vi "Lab Panel V5.10.vi"() -> ()   [LabVIEW 2013] (continued)
                      tunnel: w2159 -> [w2170 w2172 _]
                      tunnel: ["CHART PASS" "CYCLE PASS" "T-RISE PASS"] -> w2163
                      frame "CHART TEST", Default {
                      }
                      frame "CYCLE TEST" {
                      }
                      frame "T-RISE TEST" {
                      }
                    }
                    n1123 = Increment(x=w2159) -> (x+1=w2160:dbl)
                    n1124 = Greater Or Equal?(x=w2167, y=w2160) -> (x >= y?=w2169:bool)
                    n1125 = case shown="True" w2169 {
                      tunnel: w2164 -> [w2179 _]
                      tunnel: w2163 -> [w2178 _]
                      tunnel: w2162 -> [w2177 _]
                      tunnel: w2161 -> [w2176 _]
                      frame True {
                        n1126 = stacked-sequence {
                          tunnel: w2179 -> [w2183 _]
                          tunnel: w2178 -> [w2181 w2187]
                          tunnel: w2177 -> [_ w2190]
                          tunnel: w2176 -> [w2180 _]
                          frame #0 {
                            n1127 = Build Array(w2181) -> (w2184:string[])
                            n1128 = Build Array(w2183) -> (w2182:dbl[])
                            n1129 = TDMS Write(0:w2180, 5:"TEST PASS", 7:w2184, 9:w2182) -> (15:w2186:errorcluster)  [unwired: 2 in, 3 out]
                            n1130 = local write "data file error"(w2186) -> ()
                          }
                          frame #1 {
                            n1131 = Bundle(cluster=w2190, "STATUS"=w2187) -> (w2188:T4)  [unwired: 2 in]
                            n1132 = local write "RESULT LAB02-1"(TRUE) -> ()
                            n1133 = local write "DISP LAB02-1"(w2188) -> ()
                          }
                        }
                      }
                      frame False {
                      }
                    }
                  }
                }
              }
              frame #3 {
                # "LAB02-2"
                n1134 = Less?(x=w2191, y=2) -> (x < y?=w2194:bool)
                n1135 = local read "DISP LAB02-2"() -> (w2196:T4)
                n1136 = Unbundle(w2196) -> ("STATUS"=w2197:string)  [unwired: 2 out]
                n1137 = Equal?(x=w2197, y="RUN") -> (x = y?=w2193:bool)
                n1138 = And(x=w2193, y=w2194) -> (x .and. y?=w2192:bool)
                n1139 = case shown="True" w2192 {
                  tunnel: w2196 -> [_ w2202]
                  tunnel: w2191 -> [_ w2206]
                  frame False {
                  }
                  frame True {
                    n1140 = local read "SET LAB02-2"() -> (w2208:T5)
                    n1141 = local read "TDMS LAB02-2"() -> (w2201:refnum<k34>)
                    n1142 = Unbundle(w2202) -> ("CYCLE"=w2207:dbl)  [unwired: 2 out]
                    n1143 = Unbundle(w2208) -> ("CYCLES"=w2199:dbl, "T-RISE mins"=w2205:dbl)  [unwired: 3 out]
                    n1144 = case shown="\"T-RISE TEST\"" w2206 {
                      tunnel: w2205 -> [_ _ w2215]
                      tunnel: [w2210 w2212 w2215] -> w2204
                      tunnel: w2199 -> [w2210 w2212 _]
                      tunnel: ["CHART PASS" "CYCLE PASS" "T-RISE PASS"] -> w2203
                      frame "CHART TEST", Default {
                      }
                      frame "CYCLE TEST" {
                      }
                      frame "T-RISE TEST" {
                      }
                    }
                    n1145 = Increment(x=w2199) -> (x+1=w2200:dbl)
                    n1146 = Greater Or Equal?(x=w2207, y=w2200) -> (x >= y?=w2209:bool)
                    n1147 = case shown="True" w2209 {
                      tunnel: w2204 -> [w2219 _]
                      tunnel: w2203 -> [w2218 _]
                      tunnel: w2202 -> [w2217 _]
                      tunnel: w2201 -> [w2216 _]
                      frame True {
                        n1148 = stacked-sequence {
                          tunnel: w2219 -> [w2223 _]
                          tunnel: w2218 -> [w2221 w2227]
                          tunnel: w2217 -> [_ w2230]
                          tunnel: w2216 -> [w2220 _]
                          frame #0 {
                            n1149 = Build Array(w2221) -> (w2224:string[])
                            n1150 = Build Array(w2223) -> (w2222:dbl[])
                            n1151 = TDMS Write(0:w2220, 5:"TEST PASS", 7:w2224, 9:w2222) -> (15:w2226:errorcluster)  [unwired: 2 in, 3 out]
                            n1152 = local write "data file error"(w2226) -> ()
                          }
                          frame #1 {
                            n1153 = Bundle(cluster=w2230, "STATUS"=w2227) -> (w2228:T4)  [unwired: 2 in]
                            n1154 = local write "RESULT LAB02-2"(TRUE) -> ()
                            n1155 = local write "DISP LAB02-2"(w2228) -> ()
                          }
                        }
                      }
                      frame False {
                      }
                    }
                  }
                }
              }
              frame #4 {
                # "LAB03-1"
                n1156 = Less?(x=w2231, y=2) -> (x < y?=w2234:bool)
                n1157 = local read "DISP LAB03-1"() -> (w2236:T4)
                n1158 = Unbundle(w2236) -> ("STATUS"=w2237:string)  [unwired: 2 out]
                n1159 = Equal?(x=w2237, y="RUN") -> (x = y?=w2233:bool)
                n1160 = And(x=w2233, y=w2234) -> (x .and. y?=w2232:bool)
                n1161 = case shown="True" w2232 {
                  tunnel: w2236 -> [_ w2242]
                  tunnel: w2231 -> [_ w2246]
                  frame False {
                  }
                  frame True {
                    n1162 = local read "SET LAB03-1"() -> (w2248:T5)
                    n1163 = local read "TDMS LAB03-1"() -> (w2241:refnum<k34>)
                    n1164 = Unbundle(w2242) -> ("CYCLE"=w2247:dbl)  [unwired: 2 out]
                    n1165 = Unbundle(w2248) -> ("CYCLES"=w2239:dbl, "T-RISE mins"=w2245:dbl)  [unwired: 3 out]
                    n1166 = case shown="\"T-RISE TEST\"" w2246 {
                      tunnel: w2245 -> [_ _ w2255]
                      tunnel: [w2250 w2252 w2255] -> w2244
                      tunnel: w2239 -> [w2250 w2252 _]
                      tunnel: ["CHART PASS" "CYCLE PASS" "T-RISE PASS"] -> w2243
                      frame "CHART TEST", Default {
                      }
                      frame "CYCLE TEST" {
                      }
                      frame "T-RISE TEST" {
                      }
                    }
                    n1167 = Increment(x=w2239) -> (x+1=w2240:dbl)
                    n1168 = Greater Or Equal?(x=w2247, y=w2240) -> (x >= y?=w2249:bool)
                    n1169 = case shown="True" w2249 {
                      tunnel: w2244 -> [w2259 _]
                      tunnel: w2243 -> [w2258 _]
                      tunnel: w2242 -> [w2257 _]
                      tunnel: w2241 -> [w2256 _]
                      frame True {
                        n1170 = stacked-sequence {
                          tunnel: w2259 -> [w2263 _]
                          tunnel: w2258 -> [w2261 w2267]
                          tunnel: w2257 -> [_ w2270]
                          tunnel: w2256 -> [w2260 _]
                          frame #0 {
                            n1171 = Build Array(w2261) -> (w2264:string[])
                            n1172 = Build Array(w2263) -> (w2262:dbl[])
                            n1173 = TDMS Write(0:w2260, 5:"TEST PASS", 7:w2264, 9:w2262) -> (15:w2266:errorcluster)  [unwired: 2 in, 3 out]
                            n1174 = local write "data file error"(w2266) -> ()
                          }
                          frame #1 {
                            n1175 = Bundle(cluster=w2270, "STATUS"=w2267) -> (w2268:T4)  [unwired: 2 in]
                            n1176 = local write "RESULT LAB03-1"(TRUE) -> ()
                            n1177 = local write "DISP LAB03-1"(w2268) -> ()
                          }
                        }
                      }
                      frame False {
                      }
                    }
                  }
                }
              }
              frame #5 {
                # "LAB03-2"
                n1178 = Less?(x=w2271, y=2) -> (x < y?=w2274:bool)
                n1179 = local read "DISP LAB03-2"() -> (w2276:T4)
                n1180 = Unbundle(w2276) -> ("STATUS"=w2277:string)  [unwired: 2 out]
                n1181 = Equal?(x=w2277, y="RUN") -> (x = y?=w2273:bool)
                n1182 = And(x=w2273, y=w2274) -> (x .and. y?=w2272:bool)
                n1183 = case shown="True" w2272 {
                  tunnel: w2276 -> [_ w2282]
                  tunnel: w2271 -> [_ w2286]
                  frame False {
                  }
                  frame True {
                    n1184 = local read "SET LAB03-2"() -> (w2288:T5)
                    n1185 = local read "TDMS LAB03-2"() -> (w2281:refnum<k34>)
                    n1186 = Unbundle(w2282) -> ("CYCLE"=w2287:dbl)  [unwired: 2 out]
                    n1187 = Unbundle(w2288) -> ("CYCLES"=w2279:dbl, "T-RISE mins"=w2285:dbl)  [unwired: 3 out]
                    n1188 = case shown="\"T-RISE TEST\"" w2286 {
                      tunnel: w2285 -> [_ _ w2295]
                      tunnel: [w2290 w2292 w2295] -> w2284
                      tunnel: w2279 -> [w2290 w2292 _]
                      tunnel: ["CHART PASS" "CYCLE PASS" "T-RISE PASS"] -> w2283
                      frame "CHART TEST", Default {
                      }
                      frame "CYCLE TEST" {
                      }
                      frame "T-RISE TEST" {
                      }
                    }
                    n1189 = Increment(x=w2279) -> (x+1=w2280:dbl)
                    n1190 = Greater Or Equal?(x=w2287, y=w2280) -> (x >= y?=w2289:bool)
                    n1191 = case shown="True" w2289 {
                      tunnel: w2284 -> [w2299 _]
                      tunnel: w2283 -> [w2298 _]
                      tunnel: w2282 -> [w2297 _]
                      tunnel: w2281 -> [w2296 _]
                      frame True {
                        n1192 = stacked-sequence {
                          tunnel: w2299 -> [w2303 _]
                          tunnel: w2298 -> [w2301 w2307]
                          tunnel: w2297 -> [_ w2310]
                          tunnel: w2296 -> [w2300 _]
                          frame #0 {
                            n1193 = Build Array(w2301) -> (w2304:string[])
                            n1194 = Build Array(w2303) -> (w2302:dbl[])
                            n1195 = TDMS Write(0:w2300, 5:"TEST PASS", 7:w2304, 9:w2302) -> (15:w2306:errorcluster)  [unwired: 2 in, 3 out]
                            n1196 = local write "data file error"(w2306) -> ()
                          }
                          frame #1 {
                            n1197 = Bundle(cluster=w2310, "STATUS"=w2307) -> (w2308:T4)  [unwired: 2 in]
                            n1198 = local write "RESULT LAB03-2"(TRUE) -> ()
                            n1199 = local write "DISP LAB03-2"(w2308) -> ()
                          }
                        }
                      }
                      frame False {
                      }
                    }
                  }
                }
              }
              frame #6 {
                # "LAB04-1"
                n1200 = Less?(x=w2311, y=2) -> (x < y?=w2314:bool)
                n1201 = local read "DISP LAB04-1"() -> (w2316:T4)
                n1202 = Unbundle(w2316) -> ("STATUS"=w2317:string)  [unwired: 2 out]
                n1203 = Equal?(x=w2317, y="RUN") -> (x = y?=w2313:bool)
                n1204 = And(x=w2313, y=w2314) -> (x .and. y?=w2312:bool)
                n1205 = case shown="True" w2312 {
                  tunnel: w2316 -> [_ w2322]
                  tunnel: w2311 -> [_ w2326]
                  frame False {
                  }
                  frame True {
                    n1206 = local read "SET LAB04-1"() -> (w2328:T5)
                    n1207 = local read "TDMS LAB04-1"() -> (w2321:refnum<k34>)
                    n1208 = Unbundle(w2322) -> ("CYCLE"=w2327:dbl)  [unwired: 2 out]
                    n1209 = Unbundle(w2328) -> ("CYCLES"=w2319:dbl, "T-RISE mins"=w2325:dbl)  [unwired: 3 out]
                    n1210 = case shown="\"T-RISE TEST\"" w2326 {
                      tunnel: w2325 -> [_ _ w2335]
                      tunnel: [w2330 w2332 w2335] -> w2324
                      tunnel: w2319 -> [w2330 w2332 _]
                      tunnel: ["CHART PASS" "CYCLE PASS" "T-RISE PASS"] -> w2323
                      frame "CHART TEST", Default {
                      }
                      frame "CYCLE TEST" {
                      }
                      frame "T-RISE TEST" {
                      }
                    }
                    n1211 = Increment(x=w2319) -> (x+1=w2320:dbl)
                    n1212 = Greater Or Equal?(x=w2327, y=w2320) -> (x >= y?=w2329:bool)
                    n1213 = case shown="True" w2329 {
                      tunnel: w2324 -> [w2339 _]
                      tunnel: w2323 -> [w2338 _]
                      tunnel: w2322 -> [w2337 _]
                      tunnel: w2321 -> [w2336 _]
                      frame True {
                        n1214 = stacked-sequence {
                          tunnel: w2339 -> [w2343 _]
                          tunnel: w2338 -> [w2341 w2347]
                          tunnel: w2337 -> [_ w2350]
                          tunnel: w2336 -> [w2340 _]
                          frame #0 {
                            n1215 = Build Array(w2341) -> (w2344:string[])
                            n1216 = Build Array(w2343) -> (w2342:dbl[])
                            n1217 = TDMS Write(0:w2340, 5:"TEST PASS", 7:w2344, 9:w2342) -> (15:w2346:errorcluster)  [unwired: 2 in, 3 out]
                            n1218 = local write "data file error"(w2346) -> ()
                          }
                          frame #1 {
                            n1219 = Bundle(cluster=w2350, "STATUS"=w2347) -> (w2348:T4)  [unwired: 2 in]
                            n1220 = local write "RESULT LAB04-1"(TRUE) -> ()
                            n1221 = local write "DISP LAB04-1"(w2348) -> ()
                          }
                        }
                      }
                      frame False {
                      }
                    }
                  }
                }
              }
              frame #7 {
                # "LAB04-2"
                n1222 = Less?(x=w2351, y=2) -> (x < y?=w2354:bool)
                n1223 = local read "DISP LAB04-2"() -> (w2356:T4)
                n1224 = Unbundle(w2356) -> ("STATUS"=w2357:string)  [unwired: 2 out]
                n1225 = Equal?(x=w2357, y="RUN") -> (x = y?=w2353:bool)
                n1226 = And(x=w2353, y=w2354) -> (x .and. y?=w2352:bool)
                n1227 = case shown="True" w2352 {
                  tunnel: w2356 -> [_ w2362]
                  tunnel: w2351 -> [_ w2366]
                  frame False {
                  }
                  frame True {
                    n1228 = local read "SET LAB04-2"() -> (w2368:T5)
                    n1229 = local read "TDMS LAB04-2"() -> (w2361:refnum<k34>)
                    n1230 = Unbundle(w2362) -> ("CYCLE"=w2367:dbl)  [unwired: 2 out]
                    n1231 = Unbundle(w2368) -> ("CYCLES"=w2359:dbl, "T-RISE mins"=w2365:dbl)  [unwired: 3 out]
                    n1232 = case shown="\"T-RISE TEST\"" w2366 {
                      tunnel: w2365 -> [_ _ w2375]
                      tunnel: [w2370 w2372 w2375] -> w2364
                      tunnel: w2359 -> [w2370 w2372 _]
                      tunnel: ["CHART PASS" "CYCLE PASS" "T-RISE PASS"] -> w2363
                      frame "CHART TEST", Default {
                      }
                      frame "CYCLE TEST" {
                      }
                      frame "T-RISE TEST" {
                      }
                    }
                    n1233 = Increment(x=w2359) -> (x+1=w2360:dbl)
                    n1234 = Greater Or Equal?(x=w2367, y=w2360) -> (x >= y?=w2369:bool)
                    n1235 = case shown="True" w2369 {
                      tunnel: w2364 -> [w2379 _]
                      tunnel: w2363 -> [w2378 _]
                      tunnel: w2362 -> [w2377 _]
                      tunnel: w2361 -> [w2376 _]
                      frame True {
                        n1236 = stacked-sequence {
                          tunnel: w2379 -> [w2383 _]
                          tunnel: w2378 -> [w2381 w2387]
                          tunnel: w2377 -> [_ w2390]
                          tunnel: w2376 -> [w2380 _]
                          frame #0 {
                            n1237 = Build Array(w2381) -> (w2384:string[])
                            n1238 = Build Array(w2383) -> (w2382:dbl[])
                            n1239 = TDMS Write(0:w2380, 5:"TEST PASS", 7:w2384, 9:w2382) -> (15:w2386:errorcluster)  [unwired: 2 in, 3 out]
                            n1240 = local write "data file error"(w2386) -> ()
                          }
                          frame #1 {
                            n1241 = Bundle(cluster=w2390, "STATUS"=w2387) -> (w2388:T4)  [unwired: 2 in]
                            n1242 = local write "RESULT LAB04-2"(TRUE) -> ()
                            n1243 = local write "DISP LAB04-2"(w2388) -> ()
                          }
                        }
                      }
                      frame False {
                      }
                    }
                  }
                }
              }
              frame #8 {
                # "LAB05-1"
                n1244 = Less?(x=w2391, y=2) -> (x < y?=w2394:bool)
                n1245 = local read "DISP LAB05-1"() -> (w2396:T4)
                n1246 = Unbundle(w2396) -> ("STATUS"=w2397:string)  [unwired: 2 out]
                n1247 = Equal?(x=w2397, y="RUN") -> (x = y?=w2393:bool)
                n1248 = And(x=w2393, y=w2394) -> (x .and. y?=w2392:bool)
                n1249 = case shown="True" w2392 {
                  tunnel: w2396 -> [_ w2402]
                  tunnel: w2391 -> [_ w2406]
                  frame False {
                  }
                  frame True {
                    n1250 = local read "SET LAB05-1"() -> (w2408:T5)
                    n1251 = local read "TDMS LAB05-1"() -> (w2401:refnum<k34>)
                    n1252 = Unbundle(w2402) -> ("CYCLE"=w2407:dbl)  [unwired: 2 out]
                    n1253 = Unbundle(w2408) -> ("CYCLES"=w2399:dbl, "T-RISE mins"=w2405:dbl)  [unwired: 3 out]
                    n1254 = case shown="\"T-RISE TEST\"" w2406 {
                      tunnel: w2405 -> [_ _ w2415]
                      tunnel: [w2410 w2412 w2415] -> w2404
                      tunnel: w2399 -> [w2410 w2412 _]
                      tunnel: ["CHART PASS" "CYCLE PASS" "T-RISE PASS"] -> w2403
                      frame "CHART TEST", Default {
                      }
                      frame "CYCLE TEST" {
                      }
                      frame "T-RISE TEST" {
                      }
                    }
                    n1255 = Increment(x=w2399) -> (x+1=w2400:dbl)
                    n1256 = Greater Or Equal?(x=w2407, y=w2400) -> (x >= y?=w2409:bool)
                    n1257 = case shown="True" w2409 {
                      tunnel: w2404 -> [w2419 _]
                      tunnel: w2403 -> [w2418 _]
                      tunnel: w2402 -> [w2417 _]
                      tunnel: w2401 -> [w2416 _]
                      frame True {
                        n1258 = stacked-sequence {
                          tunnel: w2419 -> [w2423 _]
                          tunnel: w2418 -> [w2421 w2427]
                          tunnel: w2417 -> [_ w2430]
                          tunnel: w2416 -> [w2420 _]
                          frame #0 {
                            n1259 = Build Array(w2421) -> (w2424:string[])
                            n1260 = Build Array(w2423) -> (w2422:dbl[])
                            n1261 = TDMS Write(0:w2420, 5:"TEST PASS", 7:w2424, 9:w2422) -> (15:w2426:errorcluster)  [unwired: 2 in, 3 out]
                            n1262 = local write "data file error"(w2426) -> ()
                          }
                          frame #1 {
                            n1263 = Bundle(cluster=w2430, "STATUS"=w2427) -> (w2428:T4)  [unwired: 2 in]
                            n1264 = local write "RESULT LAB05-1"(TRUE) -> ()
                            n1265 = local write "DISP LAB05-1"(w2428) -> ()
                          }
                        }
                      }
                      frame False {
                      }
                    }
                  }
                }
              }
              frame #9 {
                # "LAB05-2"
                n1266 = Less?(x=w2431, y=2) -> (x < y?=w2434:bool)
                n1267 = local read "DISP LAB05-2"() -> (w2436:T4)
                n1268 = Unbundle(w2436) -> ("STATUS"=w2437:string)  [unwired: 2 out]
                n1269 = Equal?(x=w2437, y="RUN") -> (x = y?=w2433:bool)
                n1270 = And(x=w2433, y=w2434) -> (x .and. y?=w2432:bool)
                n1271 = case shown="True" w2432 {
                  tunnel: w2436 -> [_ w2442]
                  tunnel: w2431 -> [_ w2446]
                  frame False {
                  }
                  frame True {
                    n1272 = local read "SET LAB05-2"() -> (w2448:T5)
                    n1273 = local read "TDMS LAB05-2"() -> (w2441:refnum<k34>)
                    n1274 = Unbundle(w2442) -> ("CYCLE"=w2447:dbl)  [unwired: 2 out]
                    n1275 = Unbundle(w2448) -> ("CYCLES"=w2439:dbl, "T-RISE mins"=w2445:dbl)  [unwired: 3 out]
                    n1276 = case shown="\"T-RISE TEST\"" w2446 {
                      tunnel: w2445 -> [_ _ w2455]
                      tunnel: [w2450 w2452 w2455] -> w2444
                      tunnel: w2439 -> [w2450 w2452 _]
                      tunnel: ["CHART PASS" "CYCLE PASS" "T-RISE PASS"] -> w2443
                      frame "CHART TEST", Default {
                      }
                      frame "CYCLE TEST" {
                      }
                      frame "T-RISE TEST" {
                      }
                    }
                    n1277 = Increment(x=w2439) -> (x+1=w2440:dbl)
                    n1278 = Greater Or Equal?(x=w2447, y=w2440) -> (x >= y?=w2449:bool)
                    n1279 = case shown="True" w2449 {
                      tunnel: w2444 -> [w2459 _]
                      tunnel: w2443 -> [w2458 _]
                      tunnel: w2442 -> [w2457 _]
                      tunnel: w2441 -> [w2456 _]
                      frame True {
                        n1280 = stacked-sequence {
                          tunnel: w2459 -> [w2463 _]
                          tunnel: w2458 -> [w2461 w2467]
                          tunnel: w2457 -> [_ w2470]
                          tunnel: w2456 -> [w2460 _]
                          frame #0 {
                            n1281 = Build Array(w2461) -> (w2464:string[])
                            n1282 = Build Array(w2463) -> (w2462:dbl[])
                            n1283 = TDMS Write(0:w2460, 5:"TEST PASS", 7:w2464, 9:w2462) -> (15:w2466:errorcluster)  [unwired: 2 in, 3 out]
                            n1284 = local write "data file error"(w2466) -> ()
                          }
                          frame #1 {
                            n1285 = Bundle(cluster=w2470, "STATUS"=w2467) -> (w2468:T4)  [unwired: 2 in]
                            n1286 = local write "RESULT LAB05-2"(TRUE) -> ()
                            n1287 = local write "DISP LAB05-2"(w2468) -> ()
                          }
                        }
                      }
                      frame False {
                      }
                    }
                  }
                }
              }
            }
          }
          frame #5 {
            # "check if test cycles reached for temperature rise test"
            n1288 = stacked-sequence {
              tunnel: w2500 -> [_ _ _ _ _ _ _ _ _ _]
              tunnel: w2499 -> [_ _ _ _ _ _ _ _ _ _]
              tunnel: w2498 -> [_ _ _ _ _ _ _ _ _ _]
              tunnel: w2497 -> [_ _ _ _ _ _ _ _ _ _]
              tunnel: w2496 -> [_ _ _ _ _ _ _ _ _ _]
              tunnel: w2495 -> [_ _ _ _ _ _ _ _ _ _]
              tunnel: w2494 -> [_ _ _ _ _ _ _ _ _ _]
              tunnel: w2493 -> [_ _ _ _ _ _ _ _ _ _]
              tunnel: w2492 -> [_ _ _ _ _ _ _ _ _ _]
              tunnel: w2491 -> [_ _ _ _ _ _ _ _ _ _]
              tunnel: w2490 -> [w2506 _ _ _ _ _ _ _ _ _]
              tunnel: w2480 -> [w2501 _ _ _ _ _ _ _ _ _]
              tunnel: w2489 -> [_ w2532 _ _ _ _ _ _ _ _]
              tunnel: w2488 -> [_ _ w2562 _ _ _ _ _ _ _]
              tunnel: w2487 -> [_ _ _ w2592 _ _ _ _ _ _]
              tunnel: w2486 -> [_ _ _ _ w2622 _ _ _ _ _]
              tunnel: w2485 -> [_ _ _ _ _ w2652 _ _ _ _]
              tunnel: w2484 -> [_ _ _ _ _ _ w2682 _ _ _]
              tunnel: w2483 -> [_ _ _ _ _ _ _ w2712 _ _]
              tunnel: w2482 -> [_ _ _ _ _ _ _ _ w2742 _]
              tunnel: w2481 -> [_ _ _ _ _ _ _ _ _ w2772]
              tunnel: w2479 -> [_ w2531 _ _ _ _ _ _ _ _]
              tunnel: w2478 -> [_ _ w2561 _ _ _ _ _ _ _]
              tunnel: w2477 -> [_ _ _ w2591 _ _ _ _ _ _]
              tunnel: w2476 -> [_ _ _ _ w2621 _ _ _ _ _]
              tunnel: w2475 -> [_ _ _ _ _ w2651 _ _ _ _]
              tunnel: w2474 -> [_ _ _ _ _ _ w2681 _ _ _]
              tunnel: w2473 -> [_ _ _ _ _ _ _ w2711 _ _]
              tunnel: w2472 -> [_ _ _ _ _ _ _ _ w2741 _]
              tunnel: w2471 -> [_ _ _ _ _ _ _ _ _ w2771]
              frame #0 {
                # "LAB01-1"
                n1289 = Equal?(x=w2506, y=2) -> (x = y?=w2504:bool)
                n1290 = local read "DISP LAB01-1"() -> (w2507:T4)
                n1291 = Unbundle(w2507) -> ("STATUS"=w2508:string)  [unwired: 2 out]
                n1292 = Equal?(x=w2508, y="RUN") -> (x = y?=w2503:bool)
                n1293 = And(x=w2503, y=w2504) -> (x .and. y?=w2502:bool)
                n1294 = case shown="True" w2502 {
                  tunnel: w2507 -> [_ w2511]
                  tunnel: w2501 -> [_ w2514]
                  frame False {
                  }
                  frame True {
                    n1295 = local read "SET LAB01-1"() -> (w2513:T5)
                    n1296 = local read "TDMS LAB01-1"() -> (w2510:refnum<k34>)
                    n1297 = Unbundle(w2511) -> ("CYCLE"=w2515:dbl)  [unwired: 2 out]
                    n1298 = Unbundle(w2513) -> ("T-RISE mins"=w2512:dbl)  [unwired: 4 out]
                    n1299 = Greater Or Equal?(x=w2515, y=w2514) -> (x >= y?=w2516:bool)
                    n1300 = case shown="True" w2516 {
                      tunnel: w2512 -> [w2519 _]
                      tunnel: w2511 -> [w2518 _]
                      tunnel: w2510 -> [w2517 _]
                      frame True {
                        n1301 = stacked-sequence {
                          tunnel: w2519 -> [w2522 _]
                          tunnel: w2518 -> [_ w2527]
                          tunnel: w2517 -> [w2520 _]
                          frame #0 {
                            n1302 = Build Array("T-RISE") -> (w2524:string[])
                            n1303 = Build Array(w2522) -> (w2523:dbl[])
                            n1304 = TDMS Write(0:w2520, 5:"TEST PASS", 7:w2524, 9:w2523) -> (15:w2526:errorcluster)  [unwired: 2 in, 3 out]
                            n1305 = local write "data file error"(w2526) -> ()
                          }
                          frame #1 {
                            n1306 = Bundle(cluster=w2527, "STATUS"="T-RISE PASS") -> (w2529:T4)  [unwired: 2 in]
                            n1307 = local write "RESULT LAB01-1"(TRUE) -> ()
                            n1308 = local write "DISP LAB01-1"(w2529) -> ()
                          }
                        }
                      }
                      frame False {
                      }
                    }
                  }
                }
              }
              frame #1 {
                # "LAB01-2"
                n1309 = Equal?(x=w2532, y=2) -> (x = y?=w2535:bool)
                n1310 = local read "DISP LAB01-2"() -> (w2537:T4)
                n1311 = Unbundle(w2537) -> ("STATUS"=w2538:string)  [unwired: 2 out]
                n1312 = Equal?(x=w2538, y="RUN") -> (x = y?=w2534:bool)
                n1313 = And(x=w2534, y=w2535) -> (x .and. y?=w2533:bool)
                n1314 = case shown="True" w2533 {
                  tunnel: w2537 -> [_ w2541]
                  tunnel: w2531 -> [_ w2544]
                  frame False {
                  }
                  frame True {
                    n1315 = local read "SET LAB01-2"() -> (w2543:T5)
                    n1316 = local read "TDMS LAB01-2"() -> (w2540:refnum<k34>)
                    n1317 = Unbundle(w2541) -> ("CYCLE"=w2545:dbl)  [unwired: 2 out]
                    n1318 = Unbundle(w2543) -> ("T-RISE mins"=w2542:dbl)  [unwired: 4 out]
                    n1319 = Greater Or Equal?(x=w2545, y=w2544) -> (x >= y?=w2546:bool)
                    n1320 = case shown="True" w2546 {
                      tunnel: w2542 -> [w2549 _]
                      tunnel: w2541 -> [w2548 _]
                      tunnel: w2540 -> [w2547 _]
                      frame True {
                        n1321 = stacked-sequence {
                          tunnel: w2549 -> [w2552 _]
                          tunnel: w2548 -> [_ w2557]
                          tunnel: w2547 -> [w2550 _]
                          frame #0 {
                            n1322 = Build Array("T-RISE") -> (w2554:string[])
                            n1323 = Build Array(w2552) -> (w2553:dbl[])
                            n1324 = TDMS Write(0:w2550, 5:"TEST PASS", 7:w2554, 9:w2553) -> (15:w2556:errorcluster)  [unwired: 2 in, 3 out]
                            n1325 = local write "data file error"(w2556) -> ()
                          }
                          frame #1 {
                            n1326 = Bundle(cluster=w2557, "STATUS"="T-RISE PASS") -> (w2559:T4)  [unwired: 2 in]
                            n1327 = local write "RESULT LAB01-2"(TRUE) -> ()
                            n1328 = local write "DISP LAB01-2"(w2559) -> ()
                          }
                        }
                      }
                      frame False {
                      }
                    }
                  }
                }
              }
              frame #2 {
                # "LAB02-1"
                n1329 = Equal?(x=w2562, y=2) -> (x = y?=w2565:bool)
                n1330 = local read "DISP LAB02-1"() -> (w2567:T4)
                n1331 = Unbundle(w2567) -> ("STATUS"=w2568:string)  [unwired: 2 out]
                n1332 = Equal?(x=w2568, y="RUN") -> (x = y?=w2564:bool)
                n1333 = And(x=w2564, y=w2565) -> (x .and. y?=w2563:bool)
                n1334 = case shown="True" w2563 {
                  tunnel: w2567 -> [_ w2571]
                  tunnel: w2561 -> [_ w2574]
                  frame False {
                  }
                  frame True {
                    n1335 = local read "SET LAB02-1"() -> (w2573:T5)
                    n1336 = local read "TDMS LAB02-1"() -> (w2570:refnum<k34>)
                    n1337 = Unbundle(w2571) -> ("CYCLE"=w2575:dbl)  [unwired: 2 out]
                    n1338 = Unbundle(w2573) -> ("T-RISE mins"=w2572:dbl)  [unwired: 4 out]
                    n1339 = Greater Or Equal?(x=w2575, y=w2574) -> (x >= y?=w2576:bool)
                    n1340 = case shown="True" w2576 {
                      tunnel: w2572 -> [w2579 _]
                      tunnel: w2571 -> [w2578 _]
                      tunnel: w2570 -> [w2577 _]
                      frame True {
                        n1341 = stacked-sequence {
                          tunnel: w2579 -> [w2582 _]
                          tunnel: w2578 -> [_ w2587]
                          tunnel: w2577 -> [w2580 _]
                          frame #0 {
                            n1342 = Build Array("T-RISE") -> (w2584:string[])
                            n1343 = Build Array(w2582) -> (w2583:dbl[])
                            n1344 = TDMS Write(0:w2580, 5:"TEST PASS", 7:w2584, 9:w2583) -> (15:w2586:errorcluster)  [unwired: 2 in, 3 out]
                            n1345 = local write "data file error"(w2586) -> ()
                          }
                          frame #1 {
                            n1346 = Bundle(cluster=w2587, "STATUS"="T-RISE PASS") -> (w2589:T4)  [unwired: 2 in]
                            n1347 = local write "RESULT LAB02-1"(TRUE) -> ()
                            n1348 = local write "DISP LAB02-1"(w2589) -> ()
                          }
                        }
                      }
                      frame False {
                      }
                    }
                  }
                }
              }
              frame #3 {
                # "LAB02-2"
                n1349 = Equal?(x=w2592, y=2) -> (x = y?=w2595:bool)
                n1350 = local read "DISP LAB02-2"() -> (w2597:T4)
                n1351 = Unbundle(w2597) -> ("STATUS"=w2598:string)  [unwired: 2 out]
                n1352 = Equal?(x=w2598, y="RUN") -> (x = y?=w2594:bool)
                n1353 = And(x=w2594, y=w2595) -> (x .and. y?=w2593:bool)
                n1354 = case shown="True" w2593 {
                  tunnel: w2597 -> [_ w2601]
                  tunnel: w2591 -> [_ w2604]
                  frame False {
                  }
                  frame True {
                    n1355 = local read "SET LAB02-2"() -> (w2603:T5)
                    n1356 = local read "TDMS LAB02-2"() -> (w2600:refnum<k34>)
                    n1357 = Unbundle(w2601) -> ("CYCLE"=w2605:dbl)  [unwired: 2 out]
                    n1358 = Unbundle(w2603) -> ("T-RISE mins"=w2602:dbl)  [unwired: 4 out]
                    n1359 = Greater Or Equal?(x=w2605, y=w2604) -> (x >= y?=w2606:bool)
                    n1360 = case shown="True" w2606 {
                      tunnel: w2602 -> [w2609 _]
                      tunnel: w2601 -> [w2608 _]
                      tunnel: w2600 -> [w2607 _]
                      frame True {
                        n1361 = stacked-sequence {
                          tunnel: w2609 -> [w2612 _]
                          tunnel: w2608 -> [_ w2617]
                          tunnel: w2607 -> [w2610 _]
                          frame #0 {
                            n1362 = Build Array("T-RISE") -> (w2614:string[])
                            n1363 = Build Array(w2612) -> (w2613:dbl[])
                            n1364 = TDMS Write(0:w2610, 5:"TEST PASS", 7:w2614, 9:w2613) -> (15:w2616:errorcluster)  [unwired: 2 in, 3 out]
                            n1365 = local write "data file error"(w2616) -> ()
                          }
                          frame #1 {
                            n1366 = Bundle(cluster=w2617, "STATUS"="T-RISE PASS") -> (w2619:T4)  [unwired: 2 in]
                            n1367 = local write "RESULT LAB02-2"(TRUE) -> ()
                            n1368 = local write "DISP LAB02-2"(w2619) -> ()
                          }
                        }
                      }
                      frame False {
                      }
                    }
                  }
                }
              }
              frame #4 {
                # "LAB03-1"
                n1369 = Equal?(x=w2622, y=2) -> (x = y?=w2625:bool)
                n1370 = local read "DISP LAB03-1"() -> (w2627:T4)
                n1371 = Unbundle(w2627) -> ("STATUS"=w2628:string)  [unwired: 2 out]
                n1372 = Equal?(x=w2628, y="RUN") -> (x = y?=w2624:bool)
                n1373 = And(x=w2624, y=w2625) -> (x .and. y?=w2623:bool)
                n1374 = case shown="True" w2623 {
                  tunnel: w2627 -> [_ w2631]
                  tunnel: w2621 -> [_ w2634]
                  frame False {
                  }
                  frame True {
                    n1375 = local read "SET LAB03-1"() -> (w2633:T5)
                    n1376 = local read "TDMS LAB03-1"() -> (w2630:refnum<k34>)
                    n1377 = Unbundle(w2631) -> ("CYCLE"=w2635:dbl)  [unwired: 2 out]
                    n1378 = Unbundle(w2633) -> ("T-RISE mins"=w2632:dbl)  [unwired: 4 out]
                    n1379 = Greater Or Equal?(x=w2635, y=w2634) -> (x >= y?=w2636:bool)
                    n1380 = case shown="True" w2636 {
                      tunnel: w2632 -> [w2639 _]
                      tunnel: w2631 -> [w2638 _]
                      tunnel: w2630 -> [w2637 _]
                      frame True {
                        n1381 = stacked-sequence {
                          tunnel: w2639 -> [w2642 _]
                          tunnel: w2638 -> [_ w2647]
                          tunnel: w2637 -> [w2640 _]
                          frame #0 {
                            n1382 = Build Array("T-RISE") -> (w2644:string[])
                            n1383 = Build Array(w2642) -> (w2643:dbl[])
                            n1384 = TDMS Write(0:w2640, 5:"TEST PASS", 7:w2644, 9:w2643) -> (15:w2646:errorcluster)  [unwired: 2 in, 3 out]
                            n1385 = local write "data file error"(w2646) -> ()
                          }
                          frame #1 {
                            n1386 = Bundle(cluster=w2647, "STATUS"="T-RISE PASS") -> (w2649:T4)  [unwired: 2 in]
                            n1387 = local write "RESULT LAB03-1"(TRUE) -> ()
                            n1388 = local write "DISP LAB03-1"(w2649) -> ()
                          }
                        }
                      }
                      frame False {
                      }
                    }
                  }
                }
              }
              frame #5 {
                # "LAB03-2"
                n1389 = Equal?(x=w2652, y=2) -> (x = y?=w2655:bool)
                n1390 = local read "DISP LAB03-2"() -> (w2657:T4)
                n1391 = Unbundle(w2657) -> ("STATUS"=w2658:string)  [unwired: 2 out]
                n1392 = Equal?(x=w2658, y="RUN") -> (x = y?=w2654:bool)
                n1393 = And(x=w2654, y=w2655) -> (x .and. y?=w2653:bool)
                n1394 = case shown="True" w2653 {
                  tunnel: w2657 -> [_ w2661]
                  tunnel: w2651 -> [_ w2664]
                  frame False {
                  }
                  frame True {
                    n1395 = local read "SET LAB03-2"() -> (w2663:T5)
                    n1396 = local read "TDMS LAB03-2"() -> (w2660:refnum<k34>)
                    n1397 = Unbundle(w2661) -> ("CYCLE"=w2665:dbl)  [unwired: 2 out]
                    n1398 = Unbundle(w2663) -> ("T-RISE mins"=w2662:dbl)  [unwired: 4 out]
                    n1399 = Greater Or Equal?(x=w2665, y=w2664) -> (x >= y?=w2666:bool)
                    n1400 = case shown="True" w2666 {
                      tunnel: w2662 -> [w2669 _]
                      tunnel: w2661 -> [w2668 _]
                      tunnel: w2660 -> [w2667 _]
                      frame True {
                        n1401 = stacked-sequence {
                          tunnel: w2669 -> [w2672 _]
                          tunnel: w2668 -> [_ w2677]
                          tunnel: w2667 -> [w2670 _]
                          frame #0 {
                            n1402 = Build Array("T-RISE") -> (w2674:string[])
                            n1403 = Build Array(w2672) -> (w2673:dbl[])
                            n1404 = TDMS Write(0:w2670, 5:"TEST PASS", 7:w2674, 9:w2673) -> (15:w2676:errorcluster)  [unwired: 2 in, 3 out]
                            n1405 = local write "data file error"(w2676) -> ()
                          }
                          frame #1 {
                            n1406 = Bundle(cluster=w2677, "STATUS"="T-RISE PASS") -> (w2679:T4)  [unwired: 2 in]
                            n1407 = local write "RESULT LAB03-2"(TRUE) -> ()
                            n1408 = local write "DISP LAB03-2"(w2679) -> ()
                          }
                        }
                      }
                      frame False {
                      }
                    }
                  }
                }
              }
              frame #6 {
                # "LAB04-1"
                n1409 = Equal?(x=w2682, y=2) -> (x = y?=w2685:bool)
                n1410 = local read "DISP LAB04-1"() -> (w2687:T4)
                n1411 = Unbundle(w2687) -> ("STATUS"=w2688:string)  [unwired: 2 out]
                n1412 = Equal?(x=w2688, y="RUN") -> (x = y?=w2684:bool)
                n1413 = And(x=w2684, y=w2685) -> (x .and. y?=w2683:bool)
                n1414 = case shown="True" w2683 {
                  tunnel: w2687 -> [_ w2691]
                  tunnel: w2681 -> [_ w2694]
                  frame False {
                  }
                  frame True {
                    n1415 = local read "SET LAB04-1"() -> (w2693:T5)
                    n1416 = local read "TDMS LAB04-1"() -> (w2690:refnum<k34>)
                    n1417 = Unbundle(w2691) -> ("CYCLE"=w2695:dbl)  [unwired: 2 out]
                    n1418 = Unbundle(w2693) -> ("T-RISE mins"=w2692:dbl)  [unwired: 4 out]
                    n1419 = Greater Or Equal?(x=w2695, y=w2694) -> (x >= y?=w2696:bool)
                    n1420 = case shown="True" w2696 {
                      tunnel: w2692 -> [w2699 _]
                      tunnel: w2691 -> [w2698 _]
                      tunnel: w2690 -> [w2697 _]
                      frame True {
                        n1421 = stacked-sequence {
                          tunnel: w2699 -> [w2702 _]
                          tunnel: w2698 -> [_ w2707]
                          tunnel: w2697 -> [w2700 _]
                          frame #0 {
                            n1422 = Build Array("T-RISE") -> (w2704:string[])
                            n1423 = Build Array(w2702) -> (w2703:dbl[])
                            n1424 = TDMS Write(0:w2700, 5:"TEST PASS", 7:w2704, 9:w2703) -> (15:w2706:errorcluster)  [unwired: 2 in, 3 out]
                            n1425 = local write "data file error"(w2706) -> ()
                          }
                          frame #1 {
                            n1426 = Bundle(cluster=w2707, "STATUS"="T-RISE PASS") -> (w2709:T4)  [unwired: 2 in]
                            n1427 = local write "RESULT LAB04-1"(TRUE) -> ()
                            n1428 = local write "DISP LAB04-1"(w2709) -> ()
                          }
                        }
                      }
                      frame False {
                      }
                    }
                  }
                }
              }
              frame #7 {
                # "LAB04-2"
                n1429 = Equal?(x=w2712, y=2) -> (x = y?=w2715:bool)
                n1430 = local read "DISP LAB04-2"() -> (w2717:T4)
                n1431 = Unbundle(w2717) -> ("STATUS"=w2718:string)  [unwired: 2 out]
                n1432 = Equal?(x=w2718, y="RUN") -> (x = y?=w2714:bool)
                n1433 = And(x=w2714, y=w2715) -> (x .and. y?=w2713:bool)
                n1434 = case shown="True" w2713 {
                  tunnel: w2717 -> [_ w2721]
                  tunnel: w2711 -> [_ w2724]
                  frame False {
                  }
                  frame True {
                    n1435 = local read "SET LAB04-2"() -> (w2723:T5)
                    n1436 = local read "TDMS LAB04-2"() -> (w2720:refnum<k34>)
                    n1437 = Unbundle(w2721) -> ("CYCLE"=w2725:dbl)  [unwired: 2 out]
                    n1438 = Unbundle(w2723) -> ("T-RISE mins"=w2722:dbl)  [unwired: 4 out]
                    n1439 = Greater Or Equal?(x=w2725, y=w2724) -> (x >= y?=w2726:bool)
                    n1440 = case shown="True" w2726 {
                      tunnel: w2722 -> [w2729 _]
                      tunnel: w2721 -> [w2728 _]
                      tunnel: w2720 -> [w2727 _]
                      frame True {
                        n1441 = stacked-sequence {
                          tunnel: w2729 -> [w2732 _]
                          tunnel: w2728 -> [_ w2737]
                          tunnel: w2727 -> [w2730 _]
                          frame #0 {
                            n1442 = Build Array("T-RISE") -> (w2734:string[])
                            n1443 = Build Array(w2732) -> (w2733:dbl[])
                            n1444 = TDMS Write(0:w2730, 5:"TEST PASS", 7:w2734, 9:w2733) -> (15:w2736:errorcluster)  [unwired: 2 in, 3 out]
                            n1445 = local write "data file error"(w2736) -> ()
                          }
                          frame #1 {
                            n1446 = Bundle(cluster=w2737, "STATUS"="T-RISE PASS") -> (w2739:T4)  [unwired: 2 in]
                            n1447 = local write "RESULT LAB04-2"(TRUE) -> ()
                            n1448 = local write "DISP LAB04-2"(w2739) -> ()
                          }
                        }
                      }
                      frame False {
                      }
                    }
                  }
                }
              }
              frame #8 {
                # "LAB05-1"
                n1449 = Equal?(x=w2742, y=2) -> (x = y?=w2745:bool)
                n1450 = local read "DISP LAB05-1"() -> (w2747:T4)
                n1451 = Unbundle(w2747) -> ("STATUS"=w2748:string)  [unwired: 2 out]
                n1452 = Equal?(x=w2748, y="RUN") -> (x = y?=w2744:bool)
                n1453 = And(x=w2744, y=w2745) -> (x .and. y?=w2743:bool)
                n1454 = case shown="True" w2743 {
                  tunnel: w2747 -> [_ w2751]
                  tunnel: w2741 -> [_ w2754]
                  frame False {
                  }
                  frame True {
                    n1455 = local read "SET LAB05-1"() -> (w2753:T5)
                    n1456 = local read "TDMS LAB05-1"() -> (w2750:refnum<k34>)
                    n1457 = Unbundle(w2751) -> ("CYCLE"=w2755:dbl)  [unwired: 2 out]
                    n1458 = Unbundle(w2753) -> ("T-RISE mins"=w2752:dbl)  [unwired: 4 out]
                    n1459 = Greater Or Equal?(x=w2755, y=w2754) -> (x >= y?=w2756:bool)
                    n1460 = case shown="True" w2756 {
                      tunnel: w2752 -> [w2759 _]
                      tunnel: w2751 -> [w2758 _]
                      tunnel: w2750 -> [w2757 _]
                      frame True {
                        n1461 = stacked-sequence {
                          tunnel: w2759 -> [w2762 _]
                          tunnel: w2758 -> [_ w2767]
                          tunnel: w2757 -> [w2760 _]
                          frame #0 {
                            n1462 = Build Array("T-RISE") -> (w2764:string[])
                            n1463 = Build Array(w2762) -> (w2763:dbl[])
                            n1464 = TDMS Write(0:w2760, 5:"TEST PASS", 7:w2764, 9:w2763) -> (15:w2766:errorcluster)  [unwired: 2 in, 3 out]
                            n1465 = local write "data file error"(w2766) -> ()
                          }
                          frame #1 {
                            n1466 = Bundle(cluster=w2767, "STATUS"="T-RISE PASS") -> (w2769:T4)  [unwired: 2 in]
                            n1467 = local write "RESULT LAB05-1"(TRUE) -> ()
                            n1468 = local write "DISP LAB05-1"(w2769) -> ()
                          }
                        }
                      }
                      frame False {
                      }
                    }
                  }
                }
              }
              frame #9 {
                # "LAB05-2"
                n1469 = Equal?(x=w2772, y=2) -> (x = y?=w2775:bool)
                n1470 = local read "DISP LAB05-2"() -> (w2777:T4)
                n1471 = Unbundle(w2777) -> ("STATUS"=w2778:string)  [unwired: 2 out]
                n1472 = Equal?(x=w2778, y="RUN") -> (x = y?=w2774:bool)
                n1473 = And(x=w2774, y=w2775) -> (x .and. y?=w2773:bool)
                n1474 = case shown="True" w2773 {
                  tunnel: w2777 -> [_ w2781]
                  tunnel: w2771 -> [_ w2784]
                  frame False {
                  }
                  frame True {
                    n1475 = local read "SET LAB05-2"() -> (w2783:T5)
                    n1476 = local read "TDMS LAB05-2"() -> (w2780:refnum<k34>)
                    n1477 = Unbundle(w2781) -> ("CYCLE"=w2785:dbl)  [unwired: 2 out]
                    n1478 = Unbundle(w2783) -> ("T-RISE mins"=w2782:dbl)  [unwired: 4 out]
                    n1479 = Greater Or Equal?(x=w2785, y=w2784) -> (x >= y?=w2786:bool)
                    n1480 = case shown="True" w2786 {
                      tunnel: w2782 -> [w2789 _]
                      tunnel: w2781 -> [w2788 _]
                      tunnel: w2780 -> [w2787 _]
                      frame True {
                        n1481 = stacked-sequence {
                          tunnel: w2789 -> [w2792 _]
                          tunnel: w2788 -> [_ w2797]
                          tunnel: w2787 -> [w2790 _]
                          frame #0 {
                            n1482 = Build Array("T-RISE") -> (w2794:string[])
                            n1483 = Build Array(w2792) -> (w2793:dbl[])
